vi "pmu_FPGA Unlocked Seconds.vi"(7 "Tick Count(mSec)":u32=9942959 caption="initial tick count(mSec)", 8 "unlocked threshold (ms)":u32=1500, 11 "PPS rising?":bool) -> (2 "unlocked seconds (s)":u32=5, 3 "locked?":bool)   [LabVIEW 2013]
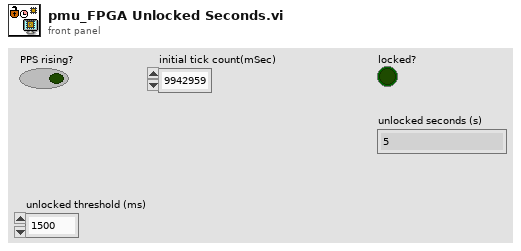
[diagram p1: front panel]
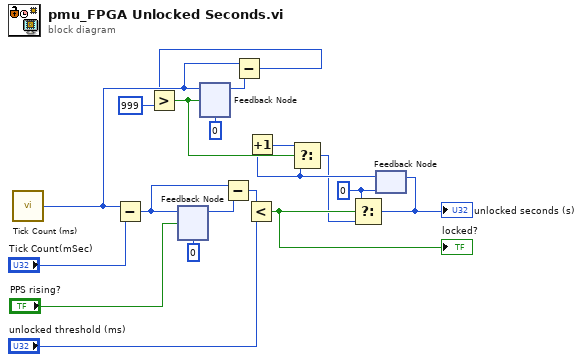
[diagram p0: block diagram]
diagram:
  w9 = u32 0 ("Unlocked Seconds")
  n1 = call "Tick Count (ms)"() -> ("Tick Count(mSec)"=w12:u32)
  n2 = Subtract(x=w12, y="Tick Count(mSec)") -> (x-y=w17:u32)
  n3 = feedback #1(u32 0 ("Tick Count(mSec)")) -> (w19:u32)
  n4 = feedback-in #1(w17, "PPS rising?") -> ()
  n5 = feedback #2(u32 0 ("Tick Count(mSec)")) -> (w13:u32)
  n6 = Subtract(x=w17, y=w19) -> (x-y=w16:u32)
  n7 = Subtract(x=w12, y=w13) -> (x-y=w3:u32)
  n8 = Greater?(x=w3, y=u32 999) -> (0:w10:bool)
  n9 = feedback-in #2(w12, w10) -> ()
  n10 = Less?(x=w16, y="unlocked threshold (ms)") -> (x < y?=w11:bool)
  "locked?" <- w11
  n11 = feedback #3(w9) -> (w7:u32)
  n12 = Increment(x=w7) -> (x+1=w8:u32)
  n13 = Select(t=w8, s=w10, f=w7) -> (s? t:f=w6:u32)
  n14 = Select(t=w9, s=w11, f=w6) -> (s? t:f=w5:u32)
  "unlocked seconds (s)" <- w5
  n15 = feedback-in #3(w5) -> ()
